vi "Read Config.vi"(8 "error in (no error)":errorcluster, 11 "Father of all uServices in":refnum<class "Father of all uServices.lvclass">) -> (0 "error out":errorcluster, 2 "TALOS.lvlib:Classes.lvlib:Config.lvclass":refnum<class "Config.lvclass">, 3 "Father of all uServices out":refnum<class "Father of all uServices.lvclass">)   [LabVIEW 2026, in "TALOS.lvlib" / "Father of all uServices.lvlib" / "Father of all uServices.lvclass"]
uses:
  Father of all uServices.lvclass
  Classes/Config/Config.lvclass
  Father of all uServices.lvclass/Father of all uServices.ctl
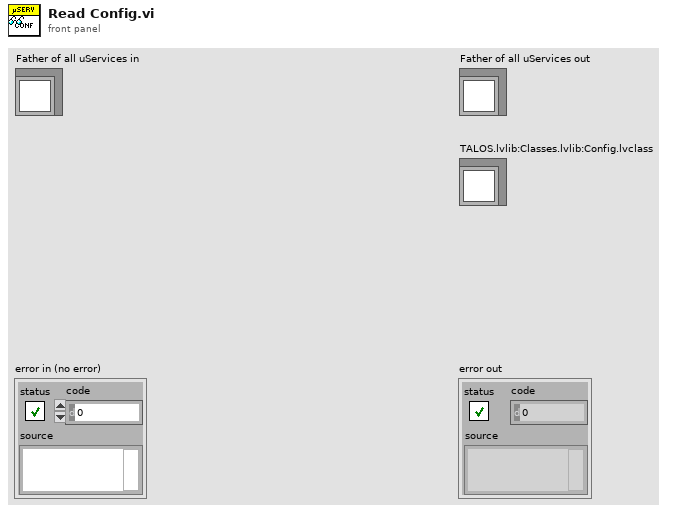
[diagram p1: front panel]
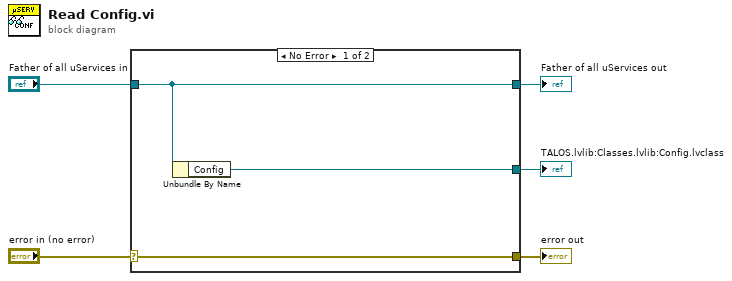
[diagram p0: block diagram]
diagram:
  n1 = case shown="No Error" "error in (no error)" {
    selector: "error in (no error)" -> [w8 w9]
    tunnel: [w8 w9] -> w4
    tunnel: [w7 w10] -> w2
    tunnel: "Father of all uServices in" -> [w7 w10]
    tunnel: [w6 _] -> w1
    frame No Error {
      n2 = Unbundle By Name(w7) -> ("Config"=w6:refnum<class "Config.lvclass">)
    }
    frame Error {
    }
  }
  "error out" <- w4
  "Father of all uServices out" <- w2
  "TALOS.lvlib:Classes.lvlib:Config.lvclass" <- w1
